vi "tm_setscanmode.vi"(8 "error in (no error)":errorcluster, 10 "Speed":u32, 11 "Handle in":u32) -> (0 "error out":errorcluster, 3 "Handle out":u32)   [LabVIEW 2011]
uses:
  tmcamcon.dll
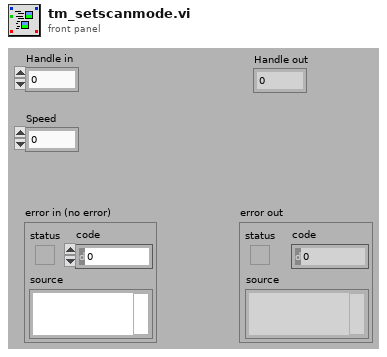
[diagram p1: front panel]
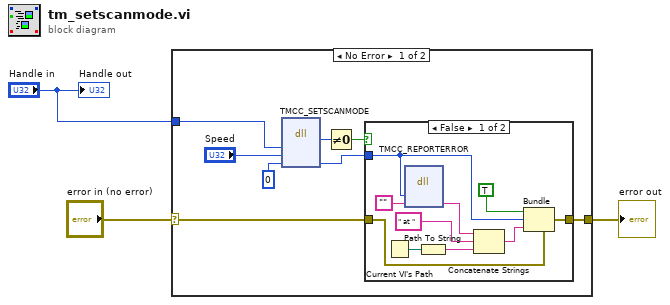
[diagram p0: block diagram]
diagram:
  n1 = case shown="No Error" "error in (no error)" {
    selector: "error in (no error)" -> [w7 w23]
    tunnel: [w6 w23] -> w2
    tunnel: "Handle in" -> [w4 _]
    frame No Error {
      n2 = dll-call lib="tmcamcon.dll" fn="TMCC_SETSCANMODE"("HDCAM"=w4, "mode"="Speed", "Erval"=0) -> ("return type"=w11:u32, "Erval"=w8:i32)  [unwired: 5 in, 2 out]
      n3 = Not Equal To 0?(x=w11) -> (x != 0?=w9:bool)
      n4 = case shown="False" w9 {
        tunnel: w7 -> [w21 w22]
        tunnel: [w20 w22] -> w6
        tunnel: w8 -> [w14 _]
        frame False {
          n5 = Current VI's Path() -> (path=w19:path)
          n6 = dll-call lib="tmcamcon.dll" fn="TMCC_REPORTERROR"("error"=w14, "buf"="") -> ("buf"=w13:string)  [unwired: 5 in, 2 out]
          n7 = Path To String(path=w19) -> (string=w15:string)
          n8 = Concatenate Strings(w13, " at ", w15) -> (w18:string)
          n9 = Bundle(cluster=w21, "status"=TRUE, "code"=w14, "source"=w18) -> (w20:errorcluster)
        }
        frame True {
        }
      }
    }
    frame Error {
    }
  }
  "error out" <- w2
  "Handle out" <- "Handle in"
